vi "BoardScreens.vi"(11 "Array 2":T1[](array[typedef])) -> ()   [LabVIEW 2015]
uses:
  <vilib>/picture/picture.llb/imagedata.ctl
panel:
  in  "Folder":path
  out "Array":picture[](array[picture])
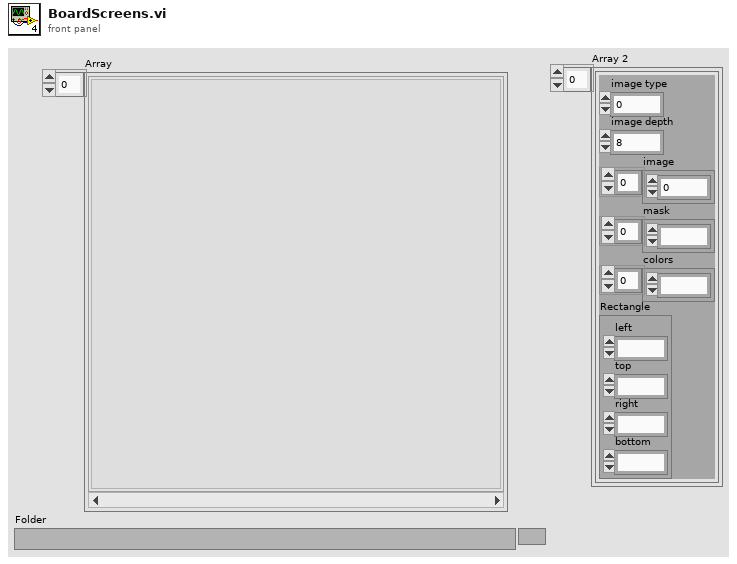
[diagram p1: front panel]
types:
  T1 = typedef "imagedata.ctl" = cluster{"image type":i32, "image depth":i32, "image":u8[], "mask":u8[], "colors":u32[], "Rectangle":cluster{"left":i16, "top":i16, "right":i16, "bottom":i16}}
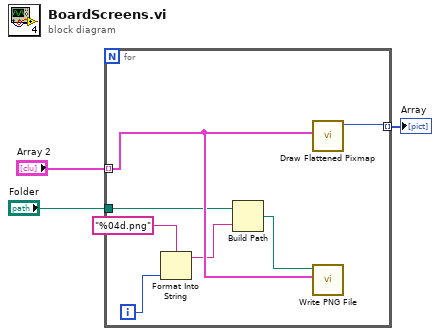
[diagram p0: block diagram]
diagram:
  n1 = for {
    tunnel: "Array 2" -> [w9] mode=indexing
    tunnel: [w10] -> w2 mode=indexing
    tunnel: "Folder" -> [w8]
    i -> [w7]
    n2 = Format Into String(format string="%04d.png", w7) -> (resulting string=w5:string)  [unwired: 2 in, 1 out]
    n3 = Build Path(base path=w8, name or relative path=w5) -> (appended path=w4:path)
    n4 = call <vilib>:"Draw Flattened Pixmap.vi"("image data"=w9) -> ("new picture"=w10:picture)  [unwired: 8 in]
    n5 = call <vilib>:"Write PNG File.vi"("image data"=w9, "path to PNG file"=w4) -> ()  [unwired: 8 in, 2 out]
  }
  "Array" <- w2
